vi "DatasetNames.vi"() -> ()   [LabVIEW 2014]
panel:
  in  "Data Types":string(combo)
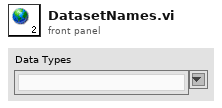
[diagram p1: front panel]
diagram:
